vi "Read BluePlotHandle.vi"(8 "error in (no error)":errorcluster, 11 "SinglePlotPanel in":refnum<class "SinglePlotPanel.lvclass">) -> (0 "error out":errorcluster, 2 "BluePlot.lvlib:BluePlotHandle.lvclass":refnum<class "BluePlotHandle.lvclass">, 3 "SinglePlotPanel out":refnum<class "SinglePlotPanel.lvclass">)   [LabVIEW 2021, in "MultiBluePlot.lvlib" / "SinglePlotPanel.lvclass"]
uses:
  SinglePlotPanel.lvclass
  SinglePlotPanel.lvclass/SinglePlotPanel.ctl
  <userlib>/Blue Origin/BluePlot (Open Source)/Classes/BluePlotHandle/BluePlotHandle.lvclass
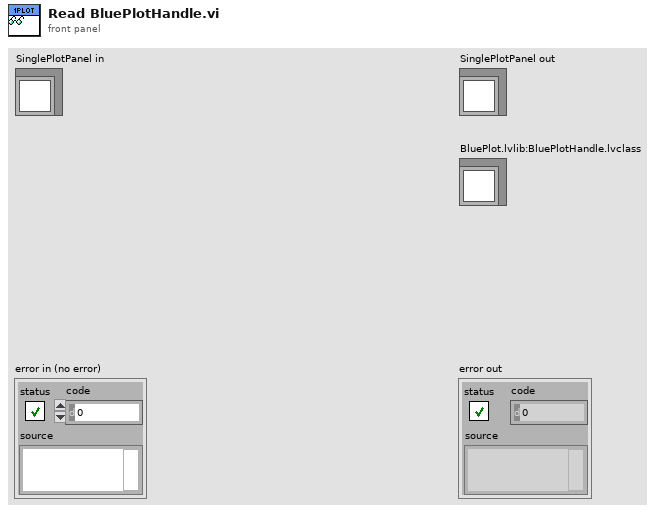
[diagram p1: front panel]
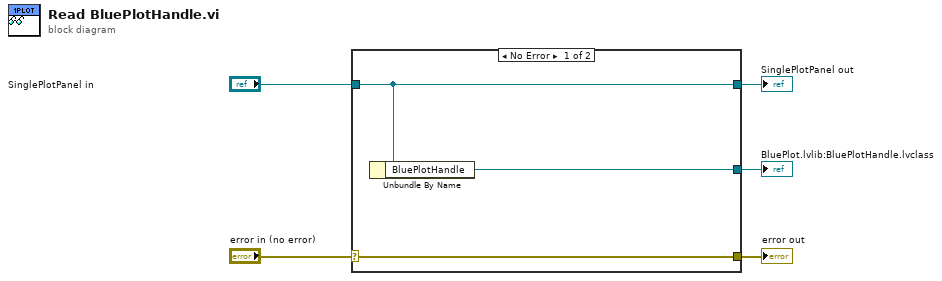
[diagram p0: block diagram]
diagram:
  n1 = case shown="No Error" "error in (no error)" {
    selector: "error in (no error)" -> [w8 w9]
    tunnel: [w8 w9] -> w4
    tunnel: [w7 w10] -> w2
    tunnel: "SinglePlotPanel in" -> [w7 w10]
    tunnel: [w6 _] -> w1
    frame No Error {
      n2 = Unbundle By Name(w7) -> ("BluePlotHandle"=w6:refnum<class "BluePlotHandle.lvclass">)
    }
    frame Error {
    }
  }
  "error out" <- w4
  "SinglePlotPanel out" <- w2
  "BluePlot.lvlib:BluePlotHandle.lvclass" <- w1
